vi "test_libssh2_sftp_shutdown.vi"() -> ()   [LabVIEW 2013, in "libssh2_integration_tests.lvlib"]
uses:
  libssh2_integration_tests.lvlib
  <vilib>/addons/_JKI Toolkits/Caraya/classes/Test/Test.lvclass
  <vilib>/addons/_JKI Toolkits/Caraya/classes/Assert/Assert.lvclass
  libssh2/libssh2.lvlib
panel:
  out "error out":errorcluster
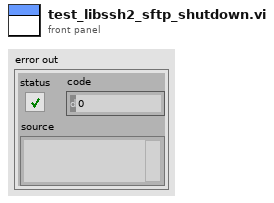
[diagram p1: front panel]
types:
  T1 = typedef "libssh2.lvlib/Session Refnum.ctl" = refnum<k1>
  T2 = typedef "libssh2.lvlib/SFTP Refnum.ctl" = refnum<k1>
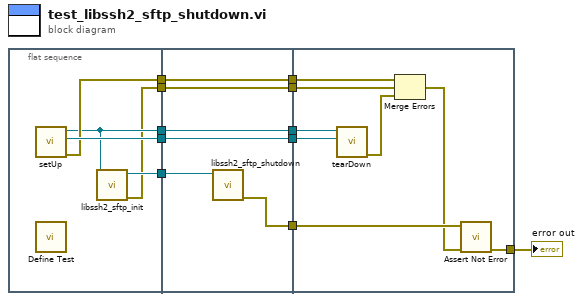
[diagram p0: block diagram]
diagram:
  n1 = flat-sequence {
    tunnel: [w13] -> w11
    tunnel: [w16] -> w10
    tunnel: [w15] -> w5
    tunnel: [w14] -> w4
    tunnel: [w12] -> w3
    tunnel: w11 -> [w22]
    tunnel: w10 -> [w21]
    tunnel: [w22] -> w9
    tunnel: [w21] -> w8
    tunnel: [w18] -> w7
    tunnel: [w20] -> w6
    tunnel: w5 -> [w20]
    tunnel: w4 -> [w19]
    tunnel: w3 -> [w17]
    tunnel: [w17] -> w2
    tunnel: w9 -> [w30]
    tunnel: w8 -> [w29]
    tunnel: w7 -> [w28]
    tunnel: w6 -> [w27]
    tunnel: w2 -> [w25]
    tunnel: [w23] -> w1
    frame #0 {
      n2 = call "setUp.vi"() -> ("error out"=w15:errorcluster, "connection ID"=w16:refnum<k5>, "session"=w13:T1)  [unwired: 9 in]
      n3 = call <vilib>:"Define Test.vi"() -> ()  [unwired: 10 in, 2 out]
      n4 = call "libssh2_sftp_init.vi"("session"=w13) -> ("error out"=w12:errorcluster, "sftp"=w14:T2)  [unwired: 9 in]
    }
    frame #1 {
      n5 = call "libssh2_sftp_shutdown.vi"("sftp"=w19) -> ("error out"=w18:errorcluster)  [unwired: 10 in]
    }
    frame #2 {
      n6 = call "tearDown.vi"("connection ID"=w29, "session"=w30) -> ("error out"=w26:errorcluster)  [unwired: 9 in]
      n7 = Merge Errors(w27, w25, w26) -> (w24:errorcluster)
      n8 = call <vilib>:"Assert Not Error.vi"("error in (no error)"=w24, "Not Error?"=w28) -> ("error out"=w23:errorcluster)  [unwired: 8 in, 1 out]
    }
  }
  "error out" <- w1
